vi "publishSettingsApplied.vi"(8 "error in (no error)":errorcluster, 11 "Model in":refnum<class "Model.lvclass">) -> (0 "error out":errorcluster, 3 "Model out":refnum<class "Model.lvclass">)   [LabVIEW 2016, in "Model.lvclass"]
uses:
  Model.lvclass
  ConfigurationTC/ConfigurationTypedefs/Set/ExampleSettings.ctl
  ComponentTemplateCore/Settings/SettingsTC/TCSettings.lvclass
  ConfigurationTC/ConfigurationTypedefs/ConfigurationTypedefs.lvlib
  ComponentTemplateCore/ComponentModel/ComponentModel/ConfigurationFileReader/ConfigurationFileReader.lvclass
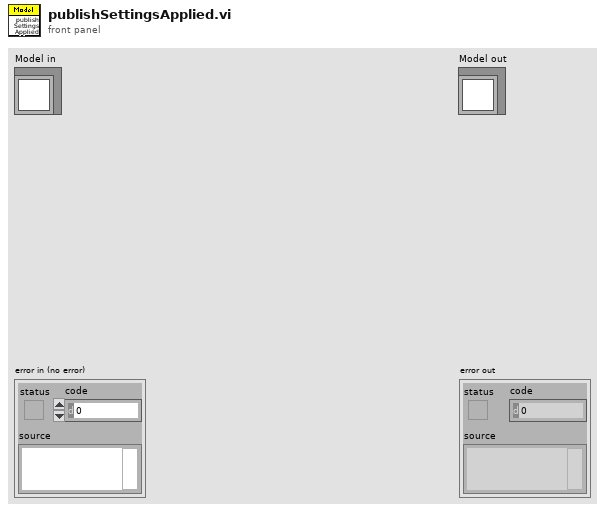
[diagram p1: front panel]
types:
  T1 = typedef "ConfigurationTypedefs.lvlib/ExampleSettings.ctl" = cluster{"exampleArray":i32[], "exampleString":string}
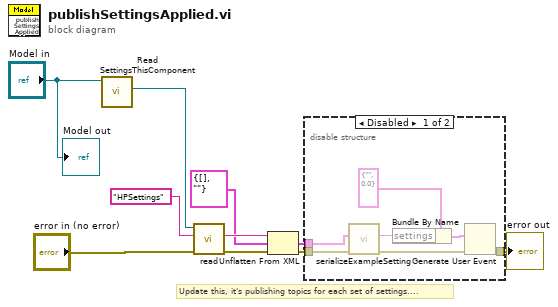
[diagram p0: block diagram]
diagram:
  # "Update this, it's publishing topics for each set of settings...."
  n1 = call-dynamic "Read SettingsThisComponent.vi"("Model in"="Model in") -> ("Settings.lvlib:TCSettings.lvclass"=w10:refnum<class "TCSettings.lvclass">)  [unwired: 8 in, 2 out]
  n2 = call-dynamic "read.vi"("error in (no error)"="error in (no error)", "Name"="HPSettings", "BaseSetting in"=w10) -> ("error out"=w4:errorcluster, "XML"=w8:string)  [unwired: 5 in, 2 out]
  n3 = Unflatten From XML(xml string=w8, type=T1 {"exampleArray"=[], "exampleString"=""} ("ExampleSettings"), error in (no error)=w4) -> (value=w6:T1, error out=w5:errorcluster)
  n4 = disable-structure shown="Disabled" {
    disable-tunnel: w6 -> [w17 _]
    disable-tunnel: w5 -> [w16 w18]
    disable-tunnel: [w15 w18] -> w1
    frame Disabled {
      n5 = call "serializeExampleSetting.vi"("error in (no error)"=w16, "ExampleSettings"=w17) -> ("error out"=w14:errorcluster, "ExampleSettings"=w12:string)  [unwired: 7 in, 1 out]
      n6 = Bundle By Name(cluster=cluster{"settings":string, "timestamp":dbl} {"settings"="", "timestamp"=0.0} ("event data"), "settings"=w12) -> (w11:cluster{"settings":string, "timestamp":dbl})
      n7 = Generate User Event(event data cluster=w11, error in=w14) -> (error out=w15:errorcluster)  [unwired: 2 in, 1 out]
    }
    frame Enabled {
    }
  }
  "error out" <- w1
  "Model out" <- "Model in"
